vi "WhenAsynchronousHelper.vi"(11 "Strings":string[](array[string])) -> ()   [LabVIEW 2011]
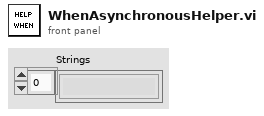
[diagram p1: front panel]
types:
  T1 = cluster{"Strings[0]":string, "Strings[1]":string, "Strings[2]":string}
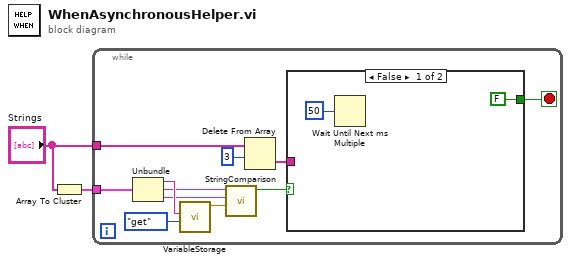
[diagram p0: block diagram]
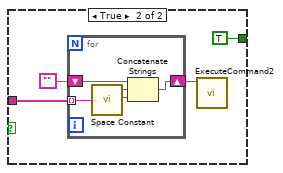
[diagram p2: hidden frame]
diagram:
  n1 = Array To Cluster(array="Strings") -> (cluster=w2:T1)
  n2 = while {
    tunnel: w2 -> [w13]
    tunnel: "Strings" -> [w5]
    stop <- w6 stop-if-true
    n3 = Unbundle(w13) -> ("Strings[0]"=w12:string, "Strings[1]"=w10:string, "Strings[2]"=w9:string)
    n4 = call "VariableStorage.vi"("menu"=enum16{"set", "get", "delete"}."get", "var name"=w12) -> ("Data Out"=w8:dbl)  [unwired: 9 in]
    n5 = call "StringComparison.vi"("cmp"=w8, "var"=w9, "op"=w10) -> ("result"=w7:bool)  [unwired: 8 in]
    n6 = Delete From Array(array=w5, length=3) -> (deleted portion=w3:string[])  [unwired: 1 in, 1 out]
    n7 = case shown="False" w7 {
      tunnel: [FALSE TRUE] -> w6
      tunnel: w3 -> [_ w18]
      frame False {
        n8 = Wait Until Next ms Multiple(millisecond multiple=u32 50) -> ()  [unwired: 1 out]
      }
      frame True {
        n9 = for {
          tunnel: w18 -> [w21] mode=indexing
          shift-right: [w23] -> w16
          shift-left: "" -> [w22]
          n10 = call <vilib>:"Space Constant.vi"() -> ("String"=w20:string)
          n11 = Concatenate Strings(w22, w21, w20) -> (w23:string)
        }
        n12 = call "ExecuteCommand2.vi"("Command"=w16) -> ()  [unwired: 11 in]
      }
    }
  }
